vi "Start Run.vi"(6 "clone#":i32, 8 "done ref":refnum<vi>, 11 "RTTarget in":refnum<class "RTTarget.lvclass">) -> (3 "RTTarget out":refnum<class "RTTarget.lvclass">)   [LabVIEW 2020, in "NI_TargetHelper.lvlib" / "RTTarget.lvclass"]
uses:
  <vilib>/TargetSupport/NI_TargetHelper/RTTarget/RTTarget.lvclass
  <vilib>/TargetSupport/NI_TargetHelper/RTTarget/RTTarget.lvclass/RTTarget.ctl
  <vilib>/TargetSupport/NI_TargetHelper/Run Target VI.ctl
  <vilib>/TargetSupport/NI_TargetHelper/NI_TargetHelper.lvlib
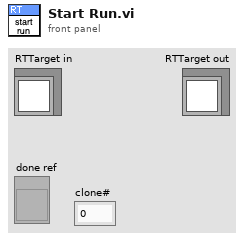
[diagram p1: front panel]
types:
  T1 = typedef "NI_TargetHelper.lvlib/Run Target VI.ctl" = refnum<vi>
  T2 = typedef "NI_TargetHelper.lvlib/Instance VIref.ctl" = refnum<vi>
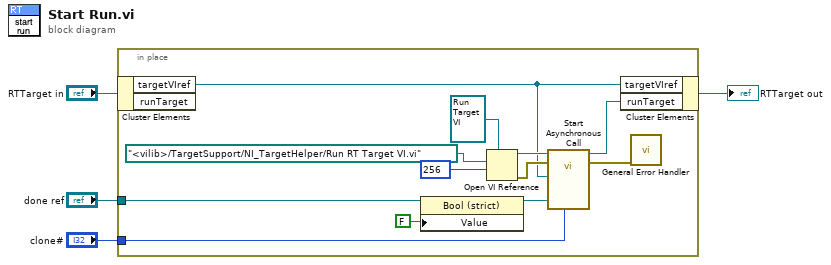
[diagram p0: block diagram]
diagram:
  n1 = in-place {
    in-place-border: "done ref" -> [w6]
    in-place-border: "clone#" -> [w5]
    n2 = in-place-cluster #1("RTTarget in") -> ("targetVIref"=w7:T2)  [unwired: 1 out]
    n3 = property class="Bool (strict)"(reference=w6, "Value"=FALSE) -> (reference out=w12:refnum<vi>)  [unwired: 1 in, 1 out]
    n4 = Open VI Reference(type specifier VI Refnum (for type only)=T1 refnum ("runTarget"), vi path=path "<vilib>/TargetSupport/NI_TargetHelper/Run RT Target VI.vi", options=256) -> (vi reference=w14:T1, error out=w10:errorcluster)  [unwired: 3 in]
    n5 = call-by-ref "Start Asynchronous Call"(reference=w14, error in=w10, "clone#"=w5, "doneRef"=w12, "targetVIref"=w7) -> (reference out=w8:T1, error out=w9:errorcluster)  [unwired: 9 in]
    n6 = in-place-cluster #1("targetVIref"=w7, "runTarget"=w8) -> (→"RTTarget out":refnum<class "RTTarget.lvclass">)
    n7 = call <vilib>:"General Error Handler.vi"("error in (no error)"=w9) -> ()  [unwired: 10 in, 5 out]
  }
